vi "Test Edit Row Functionality.vi"() -> ()   [LabVIEW 2013]
uses:
  System.Windows.Forms
  GridColumn/ColumnDefinition.ctl
  GridColumn/ColumnType.ctl
  DataTable/Edit Row (String).vi
  DataGrid.lvlib
  Events/CellValueChanged/CellValueChanged.lvclass
  Events/CellClick/CellClick.lvclass
  Events/KeyDown/KeyDown.lvclass
  DataGridView/DataGridView.lvclass
  DataTable/DataTable.lvclass
  GridColumn/GridColumn.lvclass
panel:
  in  "Edit":bool
  out "Events":string
  in  "# of Rows":i32=15
  in  "ColumnSetup":T1[](array[typedef])=[{"name"="Text", "caption"="Text", "datatype"=enum."string", "Params"="", "AutoSizeMode"=2, "FillWeight"=10.0, "MinWidth"=25, "tooltip"="Text The quick brown fox jumps over the lazy dog"}, {"name"="Details", "caption"="Details", "datatype"=enum."string", "Params"="", "AutoSizeMode"=16, "FillWeight"=100.0, "MinWidth"=150, "tooltip"="Details The quick brown fox jumps over the lazy dog"}, {"name"="Time", "caption"="", "datatype"=enum."timestamp", "Params"="", "AutoSizeMode"=1, "FillWeight"=1.0, "MinWidth"=120, "tooltip"="Time The quick brown fox jumps over the lazy dog"}, {"name"="Selection", "caption"="", "datatype"=enum."combo", "Params"="One|Two|Three", "AutoSizeMode"=6, "FillWeight"=1.0, "MinWidth"=80, "tooltip"="Selection The quick brown fox jumps over the lazy dog"}, {"name"="Function", "caption"="", "datatype"=enum."button", "Params"="", "AutoSizeMode"=6, "FillWeight"=1.0, "MinWidth"=50, "tooltip"="Function The quick brown fox jumps over the lazy dog"}, {"name"="Value", "caption"="", "datatype"=enum."numeric", "Params"="", "AutoSizeMode"=6, "FillWeight"=1.0, "MinWidth"=10, "tooltip"="Value The quick brown fox jumps over the lazy dog"}, {"name"="Active", "caption"="", "datatype"=enum."check", "Params"="", "AutoSizeMode"=6, "FillWeight"=1.0, "MinWidth"=10, "tooltip"=""}, {"name"="Status", "caption"="", "datatype"=enum."image", "Params"="", "AutoSizeMode"=6, "FillWeight"=1.0, "MinWidth"=10, "tooltip"=""}, {"name"="Link", "caption"="", "datatype"=enum."link", "Params"="", "AutoSizeMode"=1, "FillWeight"=100.0, "MinWidth"=50, "tooltip"=""}] {"MinWidth" min=2 step=1; "AutoSizeMode" items=["None"=1, "ColumnHeader"=2, "AllCellsExceptHeader"=4, "AllCells"=6, "DisplayedCellsExceptHeader"=8, "DisplayedCells"=10, "Fill"=16]; "FillWeight" min=1 max=100}
  in  "DataGridView":refnum<k24>(container)
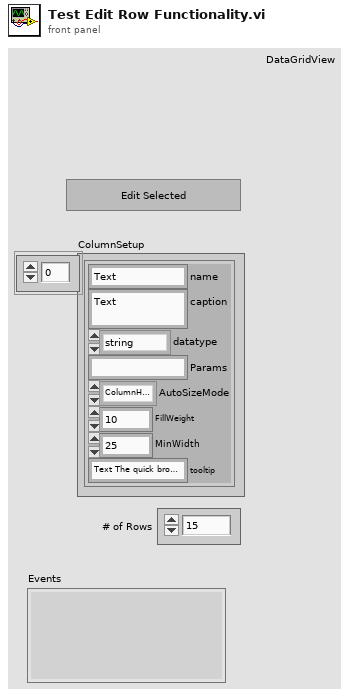
[diagram p1: front panel]
types:
  T1 = typedef "DataGrid.lvlib/GridColumn.lvclass/ColumnDefinition.ctl" = cluster{"name":string, "caption":string, "datatype":T2, "Params":string, "AutoSizeMode":i32, "FillWeight":sgl, "MinWidth":u32, "tooltip":string}
  T2 = typedef "DataGrid.lvlib/GridColumn.lvclass/ColumnType.ctl" = enum16{"string", "image", "check", "numeric", "timestamp", "button", "combo", "link"}
  T3 = cluster{"Alt":bool, "Control":bool, "KeyCode":i32, "KeyData":i32, "KeyValue":i32, "Modifiers":i32, "Shift":bool}
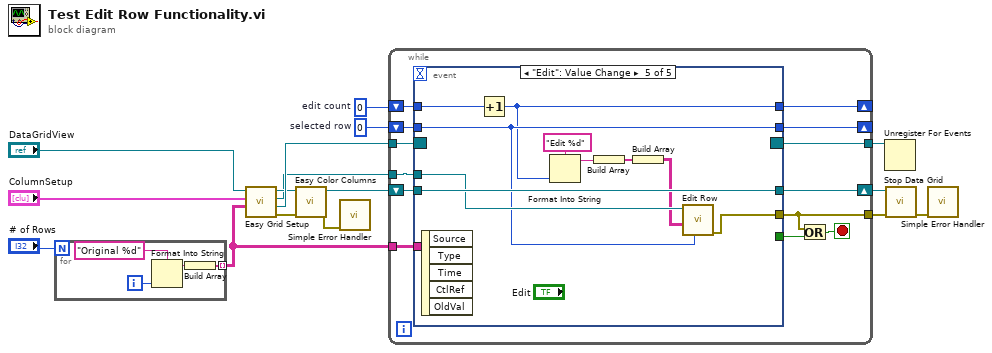
[diagram p0: block diagram]
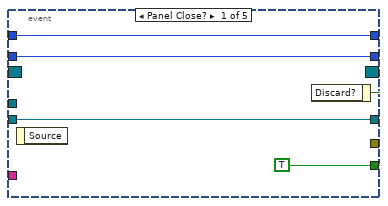
[diagram p2: hidden frame]
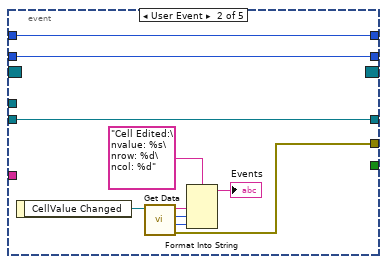
[diagram p3: hidden frame]
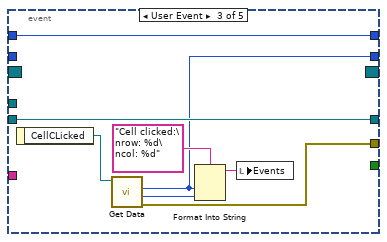
[diagram p4: hidden frame]
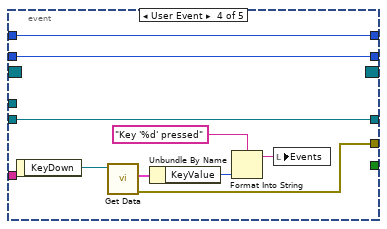
[diagram p5: hidden frame]
diagram:
  w2 = 0  # selected row
  w3 = 0  # edit count
  n1 = for {
    N: "# of Rows" -> [_]
    tunnel: [w17] -> w4 mode=indexing
    i -> [w20]
    n2 = Format Into String(format string="Original %d", w20) -> (resulting string=w18:string)  [unwired: 2 in, 1 out]
    n3 = Build Array(w18) -> (w17:string[])
  }
  n4 = call "Easy Grid Setup.vi"("DataSource Data"=w4, "ColumnSetup"="ColumnSetup", "DataGridView"="DataGridView") -> ("error out"=w13:errorcluster, "registeredEvents"=w14:refnum<event-registration>, "DataTable out"=w1:refnum<class "DataTable.lvclass">, "DataGrid out"=w12:refnum<class "DataGridView.lvclass">)  [unwired: 5 in]
  n5 = call "Easy Color Columns.vi"("error in (no error)"=w13, "DataGridView in"=w12) -> ("error out"=w9:errorcluster, "DataGridView out"=w11:refnum<class "DataGridView.lvclass">)  [unwired: 8 in]
  n6 = call <vilib>:"Simple Error Handler.vi"("error in (no error)"=w9) -> ()  [unwired: 4 in, 5 out]
  n7 = while {
    tunnel: w14 -> [w33]
    shift-right: [w31] -> w8
    shift-left: w11 -> [w32]
    tunnel: [w30] -> w10
    tunnel: w4 -> [w29]
    tunnel: [w27] -> w7
    shift-right: [w22] -> _
    shift-left: w3 -> [w23]
    shift-right: [w25] -> _
    shift-left: w2 -> [w24]
    tunnel: w1 -> [w21]
    stop <- w26 stop-if-true
    n8 = event shown="[4] \"Edit\": Value Change" {
      selector: w33 -> [_ _ _ _ _]
      dyn-events: [_ _ _ _ _] -> w30
      timeout: _ -> [_ _ _ _ _]
      tunnel: [w37 _ _ _ _] -> w28
      tunnel: w32 -> [w36 w45 w54 w64 w74]
      tunnel: [w36 w45 w54 w64 w74] -> w31
      tunnel: w29 -> [_ _ _ _ _]
      tunnel: [_ w40 w50 w58 w70] -> w27
      tunnel: [w35 w39 w49 w57 w71] -> w25
      tunnel: w24 -> [w35 w39 _ w57 w71]
      tunnel: w23 -> [w34 w38 w48 w56 w73]
      tunnel: [w34 w38 w48 w56 w68] -> w22
      tunnel: w21 -> [_ _ _ _ w72]
      event Panel Close? {
        w37 = TRUE ("Discard?")
        n9 = event-data() -> ()  [unwired: 1 in, 1 out]
        n10 = event-data("Discard?"=w37) -> ()  [unwired: 1 in, 1 out]
      }
      event User Event {
        n11 = event-data() -> ("CellValue Changed"=w44:refnum<class "Abstract EVENT.lvclass">)  [unwired: 1 in]
        n12 = call "Get Data.vi"("DataGrid.lvlib:Abstract EVENT.lvclass"=w44) -> ("error out"=w40:errorcluster, "column"=w41:i32, "row"=w42:i32, "cell value"=w43:string)  [unwired: 7 in]
        n13 = Format Into String(format string="Cell Edited:\nvalue: %s\nrow: %d\ncol: %d" ("message"), w43, w42, w41) -> (resulting string=→"Events":string)  [unwired: 2 in, 1 out]
      }
      event User Event {
        n14 = event-data() -> ("CellCLicked"=w52:refnum<class "Abstract EVENT.lvclass">)  [unwired: 1 in]
        n15 = call "Get Data.vi"("DataGrid.lvlib:Abstract EVENT.lvclass"=w52) -> ("error out"=w50:errorcluster, "column"=w51:i32, "row"=w49:i32)  [unwired: 8 in]
        n16 = Format Into String(format string="Cell clicked:\nrow: %d\ncol: %d" ("message"), w49, w51) -> (resulting string=w55:string)  [unwired: 2 in, 1 out]
        n17 = local write "Events"(w55) -> ()
      }
      event User Event {
        n18 = event-data() -> ("KeyDown"=w63:refnum<class "Abstract EVENT.lvclass">)  [unwired: 1 in]
        n19 = call "Get Data.vi"("DataGrid.lvlib:Abstract EVENT.lvclass"=w63) -> ("error out"=w58:errorcluster, "output cluster"=w60:T3)  [unwired: 9 in]
        n20 = Unbundle By Name(w60) -> ("KeyValue"=w59:i32)
        n21 = Format Into String(format string="Key '%d' pressed" ("message"), w59) -> (resulting string=w62:string)  [unwired: 2 in, 1 out]
        n22 = local write "Events"(w62) -> ()
      }
      event "Edit": Value Change {
        n23 = event-data() -> ()  [unwired: 1 in, 5 out]
        n24 = Increment(x=w73) -> (x+1=w68:i32)
        n25 = Format Into String(format string="Edit %d", w68) -> (resulting string=w67:string)  [unwired: 2 in, 1 out]
        n26 = Build Array(w67) -> (w66:string[])
        n27 = Build Array(w66) -> (w65:string[][])
        n28 = call-poly "Edit Row.vi"("Row Index"=w71, "New Row Data (or multi rows)"=w65, "DataGrid.lvlib:DataTable.lvclass 2"=w72) -> ("error out"=w70:errorcluster)  [unwired: 7 in, 1 out]
      }
    }
    n29 = Or(x=w27, y=w28) -> (x .or. y?=w26:bool)
  }
  n30 = Unregister For Events(event registration refnum=w10) -> ()  [unwired: 1 in, 1 out]
  n31 = call "Stop Data Grid.vi"("error in (no error)"=w7, "DataGridView in"=w8) -> ("error out"=w6:errorcluster)  [unwired: 8 in, 1 out]
  n32 = call <vilib>:"Simple Error Handler.vi"("error in (no error)"=w6) -> ()  [unwired: 4 in, 5 out]
